vi "HXG2_SequencerGroup.vi"(8 "error In":errorcluster, 9 "Bool Refnum":refnum<vi>, 10 "Calculated Values":T2, 11 "Analog In":T1) -> (0 "error out":errorcluster, 1 "Programmer State":T3, 2 "Running?":bool, 3 "Components Stable?":bool[](array[boolean]), 4 "Time til Step End":dbl, 5 "Current Step":i32)   [LabVIEW 2012]
uses:
  Data Types/Programmer State.ctl
  Controls/HXG2_Calculated.ctl
  Controls/HXG2_AnalogIn.ctl
  HXG2programmer.ctl
  Data Types/Programmer Execution States.ctl
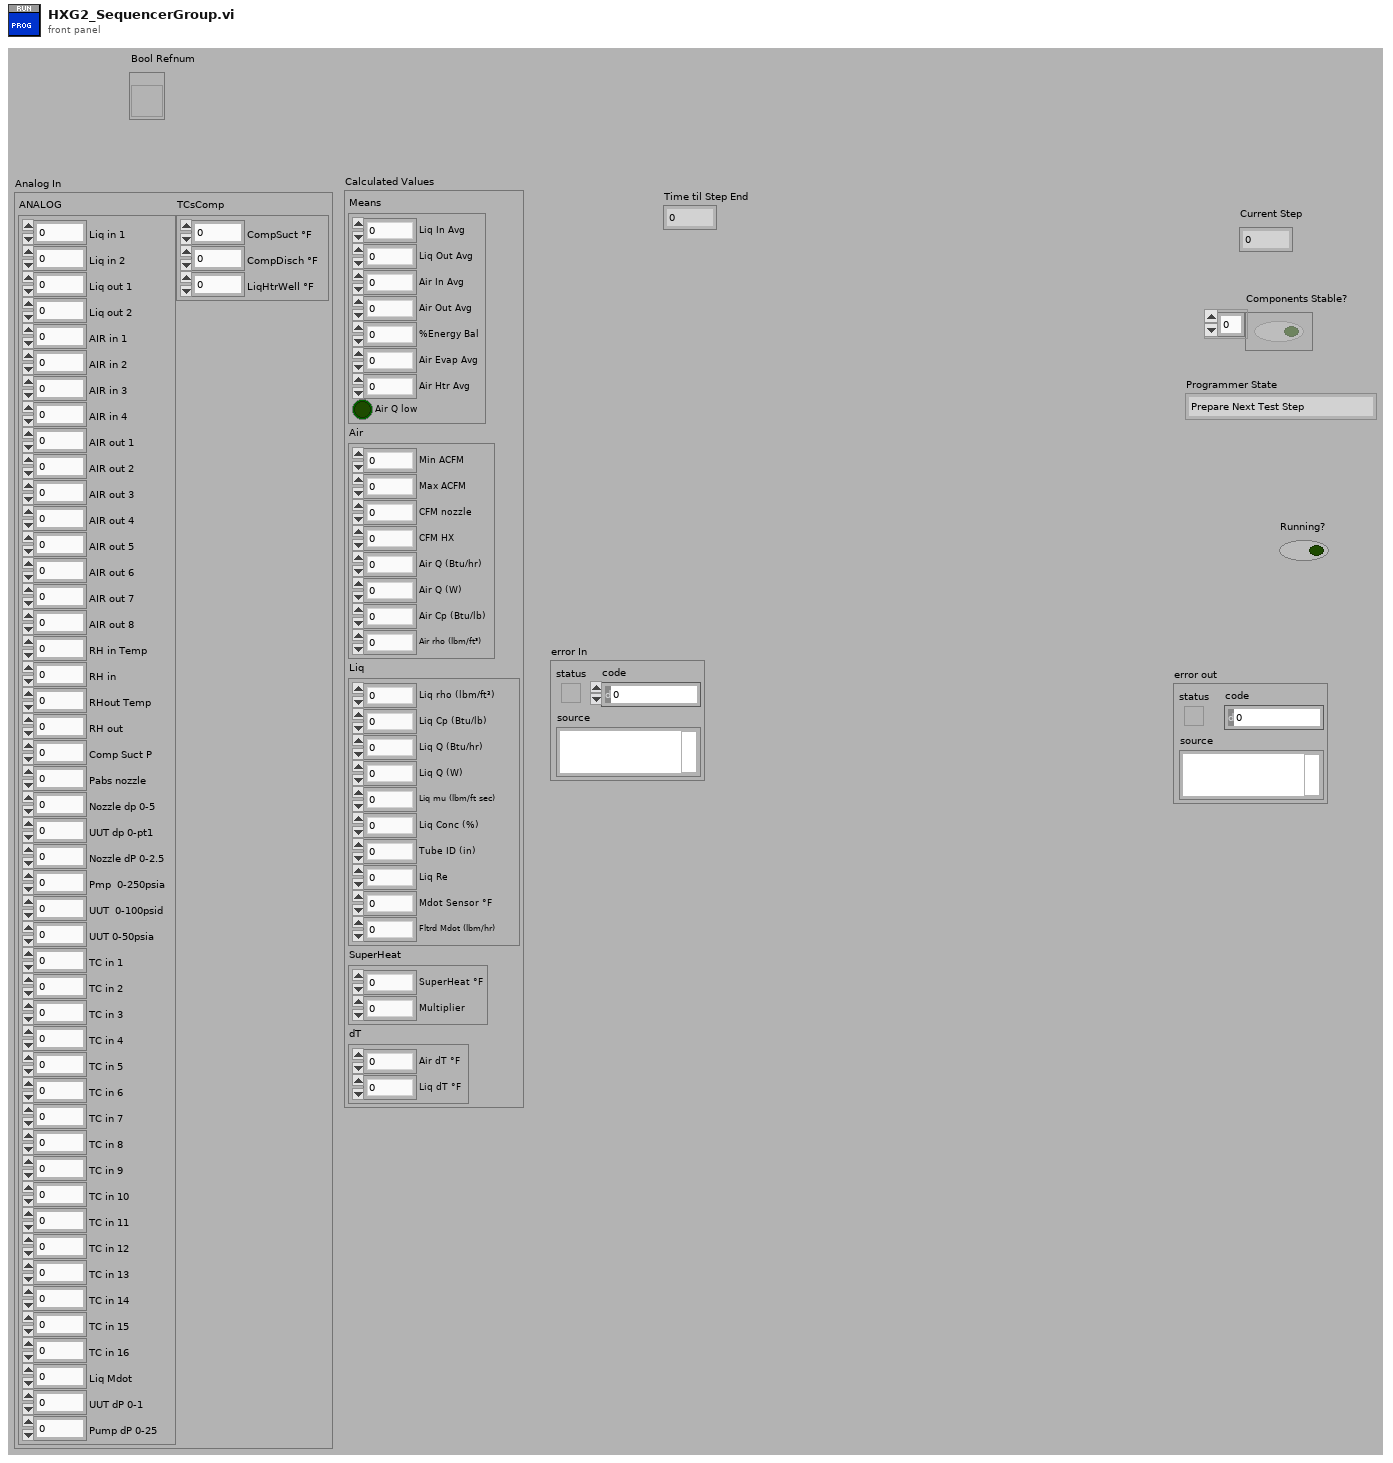
[diagram p1: front panel]
types:
  T1 = typedef "HXG2_AnalogIn.ctl" = cluster{"ANALOG":cluster{"Liq in 1":dbl, "Liq in 2":dbl, "Liq out 1":dbl, "Liq out 2":dbl, "AIR in 1":dbl, "AIR in 2":dbl, "AIR in 3":dbl, "AIR in 4":dbl, "AIR out 1":dbl, "AIR out 2":dbl, "AIR out 3":dbl, "AIR out 4":dbl, "AIR out 5":dbl, "AIR out 6":dbl, "AIR out 7":dbl, "AIR out 8":dbl, "RH in Temp":dbl, "RH in":dbl, "RHout Temp":dbl, "RH out":dbl, "Comp Suct P":dbl, "Pabs nozzle":dbl, "Nozzle dp 0-5":dbl, "UUT dp 0-pt1":dbl, "Nozzle dP 0-2.5":dbl, "Pmp  0-250psia":dbl, "UUT  0-100psid":dbl, "UUT 0-50psia":dbl, "TC in 1":dbl, "TC in 2":dbl, "TC in 3":dbl, "TC in 4":dbl, "TC in 5":dbl, "TC in 6":dbl, "TC in 7":dbl, "TC in 8":dbl, "TC in 9":dbl, "TC in 10":dbl, "TC in 11":dbl, "TC in 12":dbl, "TC in 13":dbl, "TC in 14":dbl, "TC in 15":dbl, "TC in 16":dbl, "Liq Mdot":dbl, "UUT dP 0-1":dbl, "Pump dP 0-25":dbl}, "TCsComp":cluster{"CompSuct °F  ":dbl, "CompDisch °F":dbl, "LiqHtrWell °F":dbl}}
  T2 = typedef "HXG2_Calculated.ctl" = cluster{"Means":cluster{"Liq In Avg":dbl, "Liq Out Avg":dbl, "Air In Avg":dbl, "Air Out Avg":dbl, "%Energy Bal":dbl, "Air Evap Avg":dbl, "Air Htr Avg":dbl, "Air Q low":bool}, "Air":cluster{"Min ACFM":dbl, "Max ACFM":dbl, "CFM nozzle":dbl, "CFM HX":dbl, "Air Q (Btu/hr)":dbl, "Air Q (W)":dbl, "Air Cp (Btu/lb)":dbl, "Air rho (lbm/ft³)":dbl}, "Liq":cluster{"Liq rho (lbm/ft³)":dbl, "Liq Cp (Btu/lb)":dbl, "Liq Q (Btu/hr)":dbl, "Liq Q (W)":dbl, "Liq mu (lbm/ft sec)":dbl, "Liq Conc (%)":dbl, "Tube ID (in)":dbl, "Liq Re":dbl, "Mdot Sensor °F":dbl, "Fltrd Mdot (lbm/hr)":dbl}, "SuperHeat":cluster{"SuperHeat °F":dbl, "Multiplier":dbl}, "dT":cluster{"Air dT °F":dbl, "Liq dT °F":dbl}}
  T3 = typedef "Programmer State.ctl" = enum16{"Prepare Next Test Step", "Stopped", "Running", "Stabilizing"}
  T4 = typedef "HXG2programmer.ctl" = enum16{"Write Refs", "Write Selec", "Write All", "Pass All", "React", "Write Path"}
  T5 = typedef "HXG2programmerUserSelections.ctl" = cluster{"Run Prog":bool, "Done Stop":bool, "Load Profile":bool, "Save Profile":bool, "Repeat Execution:":i32, "Start Programmer":bool, "Stop Programmer":bool}
  T6 = typedef "Programmer Step.ctl" = cluster{"Airflow (CFM)":T7, "Air Temp (°F)":T7, "Glycol Flow (lbm/hr)":T7, "Glycol Temp (°F)":T7, "Hold Time (min)":dbl, "Stability Test Time (min)":dbl, "Stability Timeout (min)":dbl, "Defrost?":bool}
  T7 = typedef "Programmer Step References.ctl" = cluster{"Setpoint":dbl, "Stability Range (±)":dbl}
  T8 = typedef "Programmer Execution States.ctl" = enum16{"Register Steps", "Initialize", "Start Test Sequence", "Register Data", "Execute Programmer", "Set Number of Repetitions", "Get Current Step Index", "Get Time Until Step Ends"}
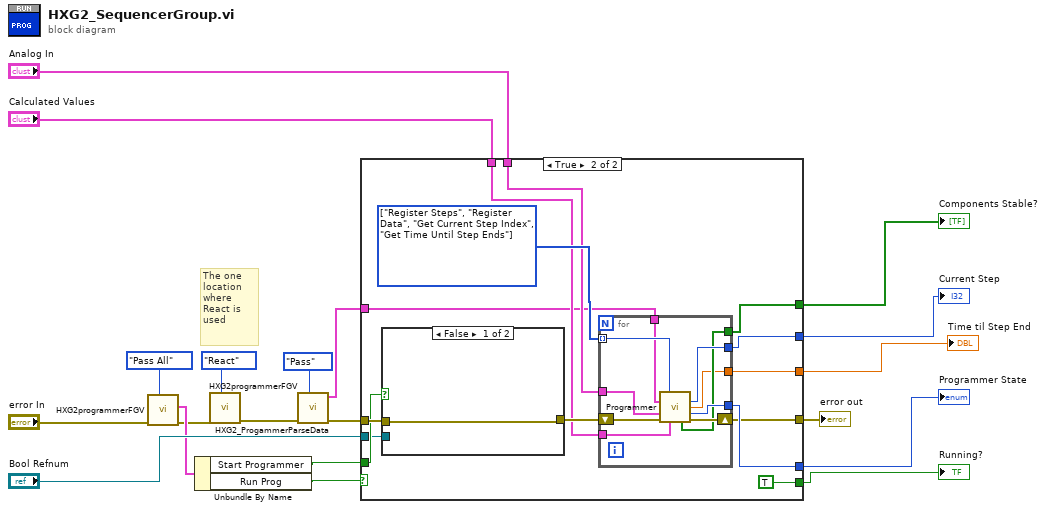
[diagram p0: block diagram]
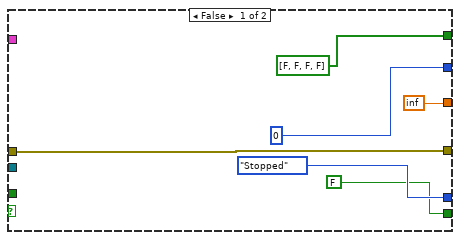
[diagram p2: hidden frame]
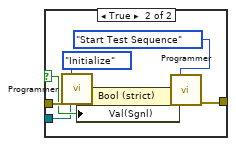
[diagram p3: hidden frame]
diagram:
  # "The one location where\nReact is used"
  n1 = call "HXG2programmerFGV.vi"("Programmer Ctrl"=HXG2programmer."Pass All", "error in (no error)"="error In") -> ("error out"=w7:errorcluster, "User Selections Out"=w10:T5)  [unwired: 5 in, 3 out]
  n2 = Unbundle By Name(w10) -> ("Start Programmer"=w2:bool, "Run Prog"=w9:bool)
  n3 = call "HXG2programmerFGV.vi"("Programmer Ctrl"=HXG2programmer."React", "error in (no error)"=w7) -> ("error out"=w6:errorcluster)  [unwired: 5 in, 4 out]
  n4 = call "HXG2_ProgammerParseData.vi"("Parse Ctrl"=enum16{"Write", "Pass"}."Pass", "error in (no error)"=w6) -> ("error out"=w5:errorcluster, "Step Array Out"=w3:T6[])  [unwired: 8 in]
  n5 = case shown="True" w9 {
    tunnel: w5 -> [w22 w39]
    tunnel: "Analog In" -> [_ w32]
    tunnel: "Calculated Values" -> [_ w33]
    tunnel: [w22 w29] -> w19
    tunnel: [0 ("Current Step") w34] -> w20
    tunnel: [Programmer_State."Stopped" ("Programmer State 2") w35] -> w16
    tunnel: [FALSE TRUE] -> w18
    tunnel: [bool[] [FALSE, FALSE, FALSE, FALSE] ("Components Stable?") w30] -> w17
    tunnel: w3 -> [_ w31]
    tunnel: w2 -> [_ w38]
    tunnel: "Bool Refnum" -> [_ w28]
    tunnel: [inf w27] -> w1
    frame False {
    }
    frame True {
      w37 = T8[] [enum."Register Steps", enum."Register Data", enum."Get Current Step Index", enum."Get Time Until Step Ends"] items=["Register Steps", "Initialize", "Start Test Sequence", "Register Data", "Execute Programmer", "Set Number of Repetitions", "Get Current Step Index", "Get Time Until Step Ends"]
      n6 = case shown="False" w38 {
        selector: w38 -> [_ w43]
        tunnel: w39 -> [w41 w49]
        tunnel: [w41 w47] -> w36
        tunnel: w28 -> [_ w42]
        frame False {
        }
        frame True {
          n7 = call "Programmer.vi"("Action"=Programmer_Execution_States."Initialize", "error in (no error)"=w49) -> ("error out"=w45:errorcluster)  [unwired: 6 in, 7 out]
          n8 = property on="Property Node" class="Bool (strict)"(reference=w42, error in=w45, "Val(Sgnl)"=w43) -> (error out=w44:errorcluster)  [unwired: 1 out]
          n9 = call "Programmer.vi"("Action"=Programmer_Execution_States."Start Test Sequence", "error in (no error)"=w44) -> ("error out"=w47:errorcluster)  [unwired: 6 in, 7 out]
        }
      }
      n10 = for {
        tunnel: w37 -> [w59] mode=indexing
        shift-right: [w57] -> w29
        shift-left: w36 -> [w58]
        tunnel: [w56] -> w35
        tunnel: [w55] -> w34
        tunnel: w33 -> [w54]
        tunnel: w32 -> [w53]
        tunnel: w31 -> [w52]
        tunnel: [w51] -> w30
        tunnel: [w50] -> w27
        n11 = call "Programmer.vi"("Action"=w59, "Step Array"=w52, "ANALOG In"=w53, "error in (no error)"=w58, "Calc Values In"=w54) -> ("Current Step"=w55:i32, "Time til Step End"=w50:dbl, "Programmer State"=w56:T3, "Components Stable?"=w51:bool[], "error out"=w57:errorcluster)  [unwired: 3 in, 3 out]
      }
    }
  }
  "Current Step" <- w20
  "error out" <- w19
  "Running?" <- w18
  "Components Stable?" <- w17
  "Programmer State" <- w16
  "Time til Step End" <- w1
